vi "Teardown.vi"(11 "Ex Event Actor in":refnum<class "Ex Event Actor.lvclass">) -> (3 "Ex Event Actor out":refnum<class "Ex Event Actor.lvclass">)   [LabVIEW 2021, in "Ex Event Actor.lvlib" / "Ex Event Actor.lvclass"]
uses:
  Ex Event Actor.lvclass
  Ex Event Actor.lvclass/Ex Event Actor.ctl
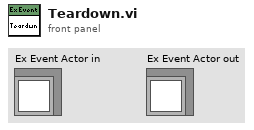
[diagram p1: front panel]
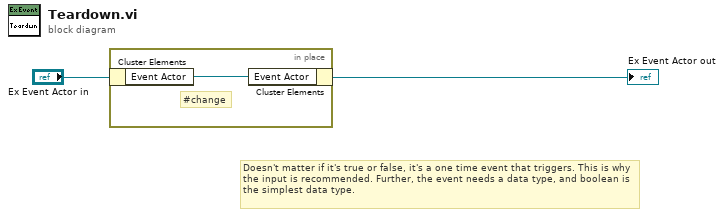
[diagram p0: block diagram]
diagram:
  # "Doesn't matter if it's true or false, it's a one time event that triggers. This is why the input is recommended. Further, the event needs a data type, and boolean is the simplest data type."
  n1 = in-place {
    # "#change"
    n2 = in-place-cluster #1("Ex Event Actor in") -> ("Event Actor"=w3:refnum<class "Event Actor.lvclass">)
    n3 = in-place-cluster #1("Event Actor"=w3) -> (→"Ex Event Actor out":refnum<class "Ex Event Actor.lvclass">)
  }
